vi "SetUpExperiment.vi"(8 "ErrorIn(No Error)":errorcluster caption="entrée d'erreur (pas d'erreur)", 10 "ScanTreeIn":refnum<vi>, 11 "Exper.lvclass":refnum<class "Experiment.lvclass">) -> (0 "sortie d'erreur":errorcluster, 3 "Exper.lvclass Out":refnum<class "Experiment.lvclass">)   [LabVIEW 2019, in "Experiment.lvclass"]
uses:
  Experiment.lvclass
  SetUpExperStates.ctl
  Experiment.lvclass/Experiment.ctl
  DevicesClass/BaseDevice/BaseDevice.lvclass
panel:
  out "MvDir(Up:T)":bool
  out "ScanTag":string
  out "CellPart":T1(ring)
  out "DblClickLine":i32
  in  "ActMeas":bool[](array[boolean])
  in  "ShowParamSuff":bool caption="Show Param. Suffix"
  in  "Param. Suffix":string
  in  "Show2ndScnParNm":bool caption="Show 2nd Scan Param. Name"
  in  "Scan Suffix":string
  in  "ShowScnSuff":bool caption="Show Scan Suffix"
  in  "Display Name":string
  in  "ShowInstrNm":bool caption="Show Instrument Name"
  in  "Before Wait(ms)":u32
  in  "ApplyWait":bool
  in  "Synch":bool
  in  "After Wait(ms)":u32
  in  "TimeMultiple(ms)":u32
  in  "RemFunc":bool
  in  "MoveFuncDown":bool
  in  "AddFunc":bool
  in  "MoveFuncUp":bool
  in  "stop":bool
  in  "FuncPannel":T2(tab)
  in  "ScanFunc":string(tree) caption="Scan Functions"
  in  "MeasFunc":i32(listbox) caption="Measurements Instruments"
  in  "HeaderFunc":i32(listbox) caption="Header Functions"
  in  "PanFunc":i32(listbox) caption="Functions Panels"
  in  "MenuPanels":i32(listbox)
  in  "LoadedDev":string(tree) caption="Loaded Instruments"
  # "Device Parameters"
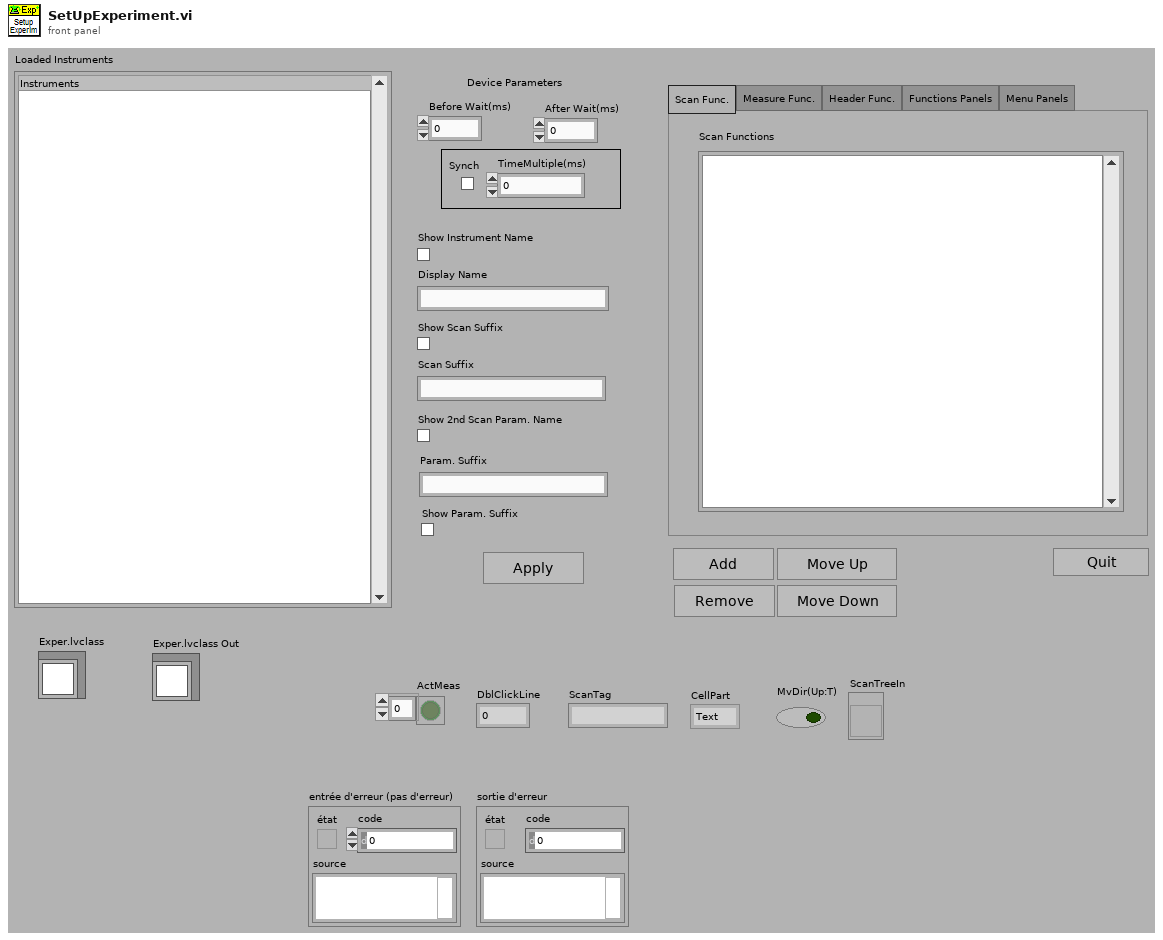
[diagram p1: front panel]
types:
  T1 = enum16{"Text", "Background", "Item Symbol", "Open/Close Symbol", "Hierarchy Lines", "Right Border", "Bottom Border", "Bottom Right Corner", "Unknown Part"}
  T2 = enum32{"Scan Func.", "Measure Func.", "Header Func.", "Functions Panels", "Menu Panels"}
  T3 = typedef "SetUpExperStates.ctl" = enum16{"InitProg", "AddScanFunc", "RmveScanFunc", "PlaceScanFunc", "NewScanTask", "MvScanFunc", "AddMeasFunc", "RmveMeasFunc", "MvMeasFuncUp", "MvMeasFuncDn", "AddHeaderFunc", "RmveHeadFunc", "MvHeadFuncUp", "MvHeadFuncDn", "AddFuncPan", "RemFuncPan", "MvFuncPanUp", "MvFuncPanDn", "AddMenuPan", "RemMenuPan", "Wait", "Stop", "DblClickMeasPan", "DblClickScanPan"}
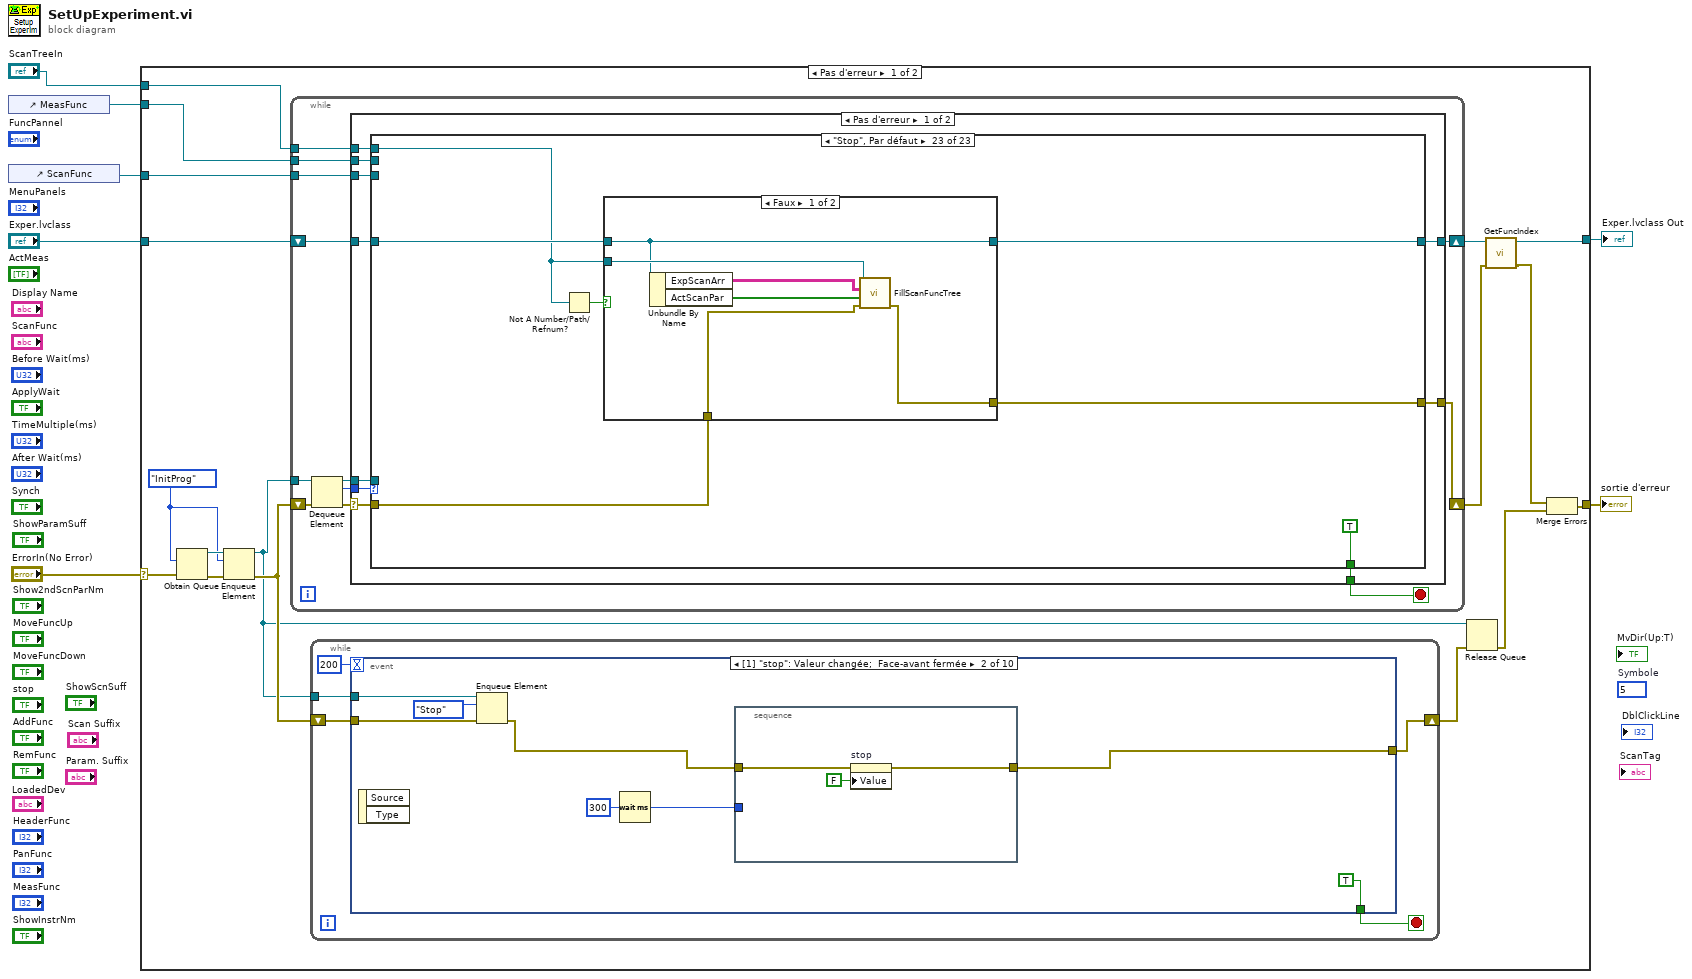
[diagram p0: block diagram]
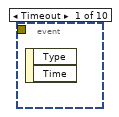
[diagram p2: hidden frame]
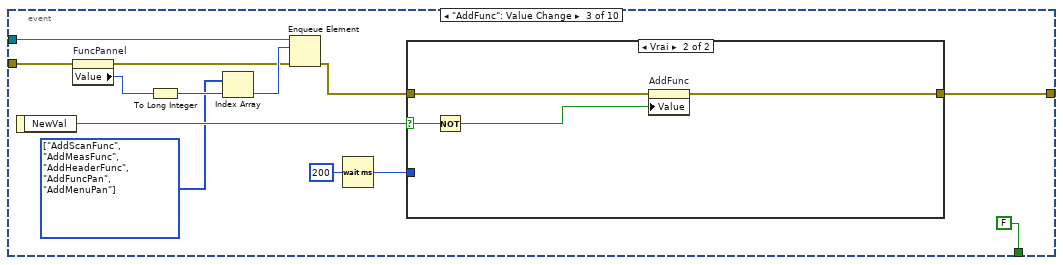
[diagram p3: hidden frame]
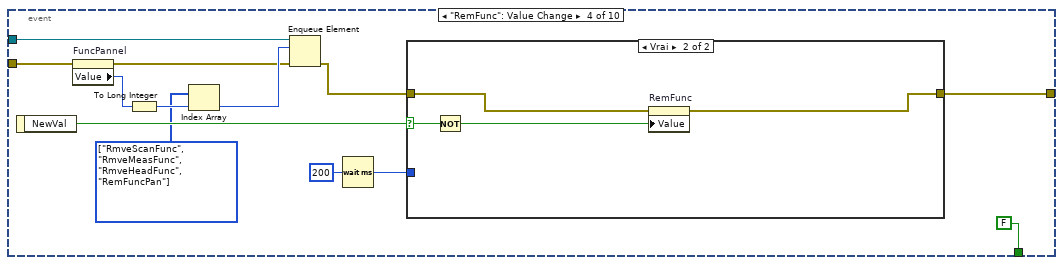
[diagram p5: hidden frame]
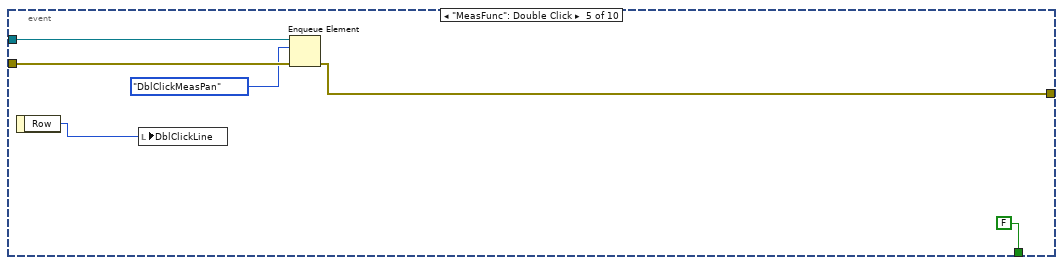
[diagram p7: hidden frame]
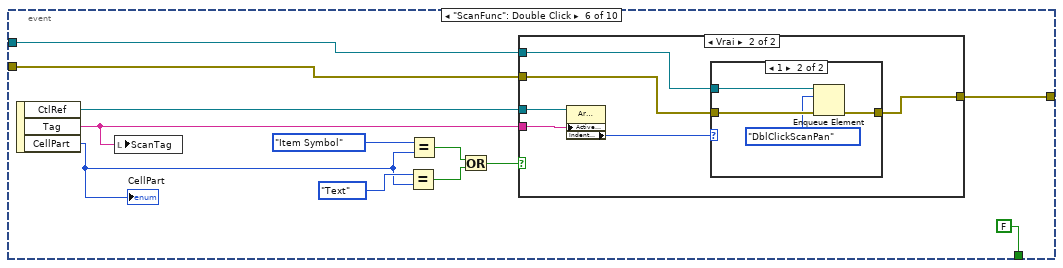
[diagram p8: hidden frame]
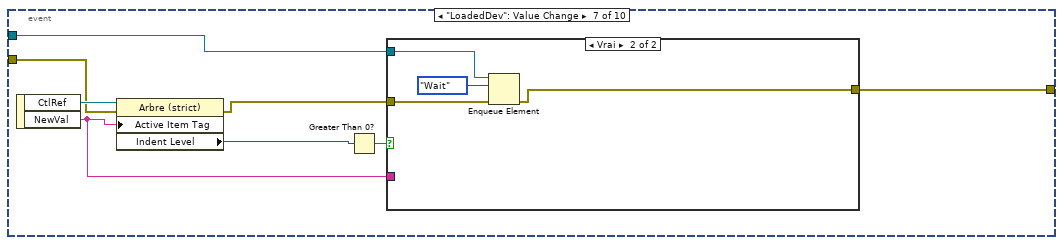
[diagram p11: hidden frame]
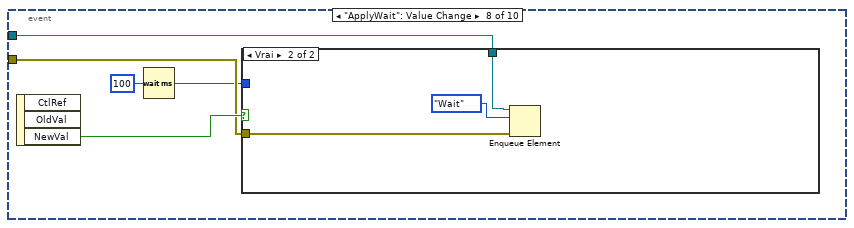
[diagram p13: hidden frame]
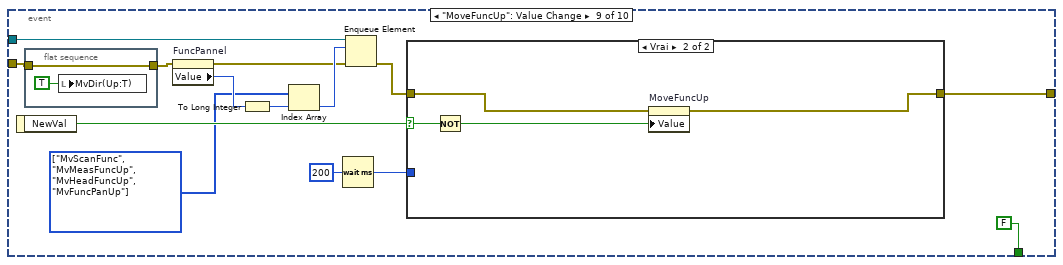
[diagram p15: hidden frame]
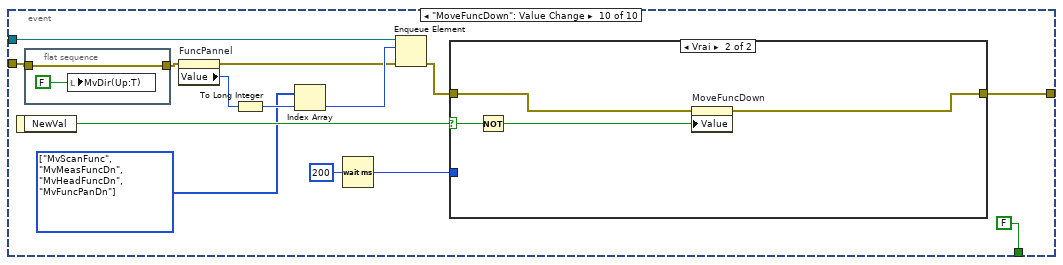
[diagram p17: hidden frame]
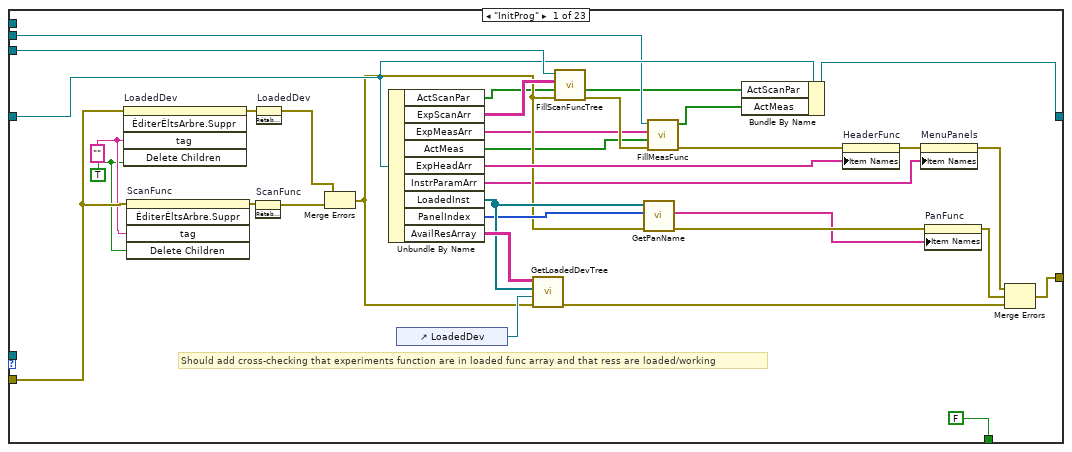
[diagram p19: hidden frame]
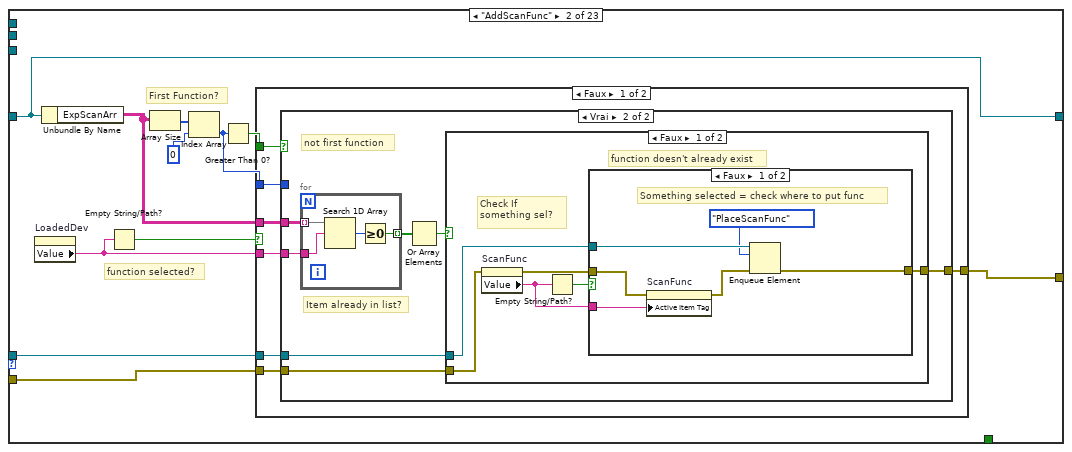
[diagram p20: hidden frame]
diagram:
  (unwired) 5  # Symbole
  n1 = control-ref of="MeasFunc"() -> (w2:refnum<vi>)
  n2 = control-ref of="ScanFunc"() -> (w5:refnum<vi>)
  n3 = case shown="Pas d'erreur" "ErrorIn(No Error)" {
    selector: "ErrorIn(No Error)" -> [w22 w1018]
    tunnel: [w12 w1018] -> w6
    tunnel: w5 -> [w18 _]
    tunnel: "Exper.lvclass" -> [w16 w1017]
    tunnel: [w10 w1017] -> w3
    tunnel: w2 -> [w9 _]
    tunnel: "ScanTreeIn" -> [w8 _]
    frame No Error {
      w21 = SetUpExperStates."InitProg" ("Énum")
      n4 = Obtain Queue(element data type=w21, error in (no error)=w22) -> (queue out=w23:refnum<queue>, error out=w24:errorcluster)  [unwired: 3 in, 1 out]
      n5 = Enqueue Element(queue=w23, element=w21, error in (no error)=w24) -> (queue out=w17:refnum<queue>, error out=w19:errorcluster)  [unwired: 1 in, 1 out]
      n6 = while {
        tunnel: w17 -> [w179]
        shift-right: [w172] -> w14
        shift-left: w19 -> [w177]
        tunnel: w18 -> [w175]
        shift-right: [w173] -> w15
        shift-left: w16 -> [w174]
        tunnel: w9 -> [w171]
        tunnel: w8 -> [w170]
        stop <- w176 stop-if-true
        n7 = Dequeue Element(queue=w179, error in (no error)=w177) -> (queue out=w178:refnum<queue>, element=w180:T3, error out=w181:errorcluster)  [unwired: 1 in, 1 out]
        n8 = case shown="Pas d'erreur" w181 {
          selector: w181 -> [w189 w1015]
          tunnel: w180 -> [w191 _]
          tunnel: w178 -> [w190 _]
          tunnel: [w188 TRUE] -> w176
          tunnel: [w187 w1015] -> w172
          tunnel: w175 -> [w186 _]
          tunnel: w174 -> [w185 w1014]
          tunnel: [w184 w1014] -> w173
          tunnel: w171 -> [w183 _]
          tunnel: w170 -> [w182 _]
          frame No Error {
            n9 = case shown="\"Stop\", Par défaut" w191 {
              tunnel: w190 -> [_ w231 _ _ _ _ _ _ _ _ _ _ _ _ _ _ _ _ _ _ _ _ _]
              tunnel: w189 -> [w206 w230 w290 w308 w390 w421 w471 w513 w536 w552 w582 w611 w646 w683 w709 w730 w763 w822 w880 w906 w936 w965 w1003]
              tunnel: [FALSE _ _ _ _ _ _ _ _ _ _ _ _ _ _ _ _ _ _ _ _ _ TRUE] -> w188
              tunnel: [w222 w234 w284 w301 w384 w418 w469 w512 w535 w546 w577 w609 w644 w682 w704 w738 w761 w820 w879 w901 w935 w961 w1001] -> w187
              tunnel: w186 -> [w218 _ w285 w299 w388 w419 _ _ _ w555 _ _ _ _ _ _ _ _ _ _ _ _ _]
              tunnel: w185 -> [w213 w226 w283 w298 w386 w417 w464 w507 w544 w557 w576 w603 w639 w677 w703 w733 w760 w819 w874 w900 w928 w957 w1004]
              tunnel: [w195 w226 w282 w297 w385 w416 w463 w506 w543 w556 w575 w602 w638 w676 w702 w732 w759 w818 w873 w899 w927 w956 w1000] -> w184
              tunnel: w183 -> [w196 _ _ _ _ _ _ w505 w539 _ w573 w599 _ _ _ _ _ _ _ _ _ _ _]
              tunnel: w182 -> [_ _ _ _ _ _ _ _ _ _ _ _ _ _ _ _ _ _ _ _ _ _ w999]
              frame "InitProg" {
                w205 = "" ("Tag")
                w204 = TRUE ("Supprimer les enfants ?")
                # "Should add cross-checking that experiments function are in loaded func array and that ress are loaded/working"
                n10 = invoke on="LoadedDev" class="Arbre (strict)" method="ÉditerÉltsArbre.Suppr"(error in=w206, "tag"=w205, "Delete Children"=w204) -> (error out=w225:errorcluster)  [unwired: 2 in, 4 out]
                n11 = invoke on="ScanFunc" class="Arbre (strict)" method="ÉditerÉltsArbre.Suppr"(error in=w206, "tag"=w205, "Delete Children"=w204) -> (error out=w221:errorcluster)  [unwired: 2 in, 4 out]
                n12 = invoke on="ScanFunc" class="Arbre (strict)" method="RétablirValParDéfaut"(error in=w221) -> (error out=w219:errorcluster)  [unwired: 2 in, 2 out]
                n13 = invoke on="LoadedDev" class="Arbre (strict)" method="RétablirValParDéfaut"(error in=w225) -> (error out=w220:errorcluster)  [unwired: 2 in, 2 out]
                n14 = Merge Errors(w220, w219) -> (w209:errorcluster)
                n15 = Unbundle By Name(w213) -> ("ActScanPar"=w193:bool[], "ExpScanArr"=w216:string[][], "ExpMeasArr"=w198:string[], "ActMeas"=w197:bool[], "ExpHeadArr"=w217:string[], "InstrParamArr"=w202:string[], "LoadedInst"=w211:refnum<class "BaseDevice.lvclass">[], "PanelIndex"=w210:i32[], "AvailResArray"=w212:string[][])
                n16 = control-ref of="LoadedDev"() -> (w215:refnum<vi>)
                n17 = call "GetLoadedDevTree.vi"("ErrorIn"=w209, "TreeRefIn"=w215, "LoadedInst"=w211, "AvailRessArray"=w212) -> ("ErrorOut"=w223:errorcluster)  [unwired: 7 in]
                n18 = call "FillScanFuncTree.vi"("ErrorIn(No Error)"=w209, "Active ScanPar"=w193, "ScanFunc"=w216, "ScanTreeRef"=w218) -> ("sortie d'erreur"=w200:errorcluster, "Active ScanParOut"=w192:bool[])  [unwired: 6 in]
                n19 = call "GetPanName.vi"("error in (no error)"=w209, "PanelIndex"=w210, "LoadedDev In"=w211) -> ("error out"=w208:errorcluster, "PanelNames"=w207:string[])  [unwired: 6 in, 1 out]
                n20 = call "FillMeasFunc.vi"("ErrorIn(No Error)"=w200, "ActMeas"=w197, "MeasFunc"=w198, "ListRef"=w196) -> ("sortie d'erreur"=w199:errorcluster, "ActMeasOut"=w194:bool[])  [unwired: 6 in]
                n21 = Bundle By Name(cluster=w213, "ActScanPar"=w192, "ActMeas"=w194) -> (w195:refnum<class "Experiment.lvclass">)
                n22 = property on="HeaderFunc" class="LstDér (strict)"(error in=w199, "Item Names"=w217) -> (error out=w203:errorcluster)  [unwired: 1 in, 1 out]
                n23 = property on="MenuPanels" class="LstDér (strict)"(error in=w203, "Item Names"=w202) -> (error out=w201:errorcluster)  [unwired: 1 in, 1 out]
                n24 = property on="PanFunc" class="LstDér (strict)"(error in=w208, "Item Names"=w207) -> (error out=w214:errorcluster)  [unwired: 1 in, 1 out]
                n25 = Merge Errors(w201, w214, w223) -> (w222:errorcluster)
              }
              frame "AddScanFunc" {
                # "function selected?"
                # "First Function?"
                n26 = property on="LoadedDev" class="Arbre (strict)"() -> ("Value"=w229:string)  [unwired: 2 in, 2 out]
                n27 = Unbundle By Name(w226) -> ("ExpScanArr"=w227:string[][])
                n28 = Empty String/Path?(string/path=w229) -> (empty?=w228:bool)
                n29 = Array Size(array=w227) -> (size(s)=w236:i32[])
                n30 = Index Array(array=w236, index=0 ("indice")) -> (element=w232:i32)
                n31 = Greater Than 0?(x=w232) -> (x > 0?=w233:bool)
                n32 = case shown="Faux" w228 {
                  tunnel: [w243 _] -> w234
                  tunnel: w233 -> [w242 _]
                  tunnel: w232 -> [w241 _]
                  tunnel: w231 -> [w240 _]
                  tunnel: w230 -> [w239 _]
                  tunnel: w227 -> [w238 _]
                  tunnel: w229 -> [w237 _]
                  frame False {
                    n33 = case shown="Vrai" w242 {
                      tunnel: [w244 w250] -> w243
                      tunnel: w241 -> [_ _]
                      tunnel: w238 -> [_ w254]
                      tunnel: w237 -> [_ w253]
                      tunnel: w240 -> [w246 w251]
                      tunnel: w239 -> [w245 w248]
                      frame False {
                        # "first function"
                        n34 = Enqueue Element(queue=w246, element=SetUpExperStates."NewScanTask" ("Énum"), error in (no error)=w245) -> (error out=w244:errorcluster)  [unwired: 1 in, 2 out]
                      }
                      frame True {
                        # "not first function"
                        # "Item already in list?"
                        n35 = for {
                          tunnel: [w275] -> w252 mode=indexing
                          tunnel: w253 -> [w274]
                          tunnel: w254 -> [w273] mode=indexing
                          n36 = Search 1D Array(1D array=w273, element=w274) -> (index of element=w276:i32)  [unwired: 1 in]
                          n37 = Greater Or Equal To 0?(x=w276) -> (x >= 0?=w275:bool)
                        }
                        n38 = Or Array Elements(Boolean array=w252) -> (logical OR=w249:bool)
                        n39 = case shown="Faux" w249 {
                          tunnel: w251 -> [w260 _]
                          tunnel: [w259 w271] -> w250
                          tunnel: w248 -> [w256 w271]
                          frame False {
                            # "function doesn't already exist"
                            # "Check If something sel?"
                            n40 = property on="ScanFunc" class="Arbre (strict)"(error in=w256) -> (error out=w255:errorcluster, "Value"=w257:string)  [unwired: 1 in, 1 out]
                            n41 = Empty String/Path?(string/path=w257) -> (empty?=w258:bool)
                            n42 = case shown="Faux" w258 {
                              tunnel: w260 -> [w266 w269]
                              tunnel: [w265 w268] -> w259
                              tunnel: w257 -> [w264 _]
                              tunnel: w255 -> [w262 w267]
                              frame False {
                                # "Something selected = check where to put func"
                                n43 = property on="ScanFunc" class="Arbre (strict)"(error in=w262, "Active Item Tag"=w264) -> (error out=w261:errorcluster)  [unwired: 1 in, 1 out]
                                n44 = Enqueue Element(queue=w266, element=SetUpExperStates."PlaceScanFunc" ("Énum"), error in (no error)=w261) -> (error out=w265:errorcluster)  [unwired: 1 in, 2 out]
                              }
                              frame True {
                                # "Nothing sel = add new Group"
                                n45 = Enqueue Element(queue=w269, element=SetUpExperStates."NewScanTask" ("Énum"), error in (no error)=w267) -> (error out=w268:errorcluster)  [unwired: 1 in, 2 out]
                              }
                            }
                          }
                          frame True {
                            # "function already exist"
                            n46 = One Button Dialog(message="Cette fonction est déjà dans la liste") -> ()  [unwired: 1 in, 1 out]
                          }
                        }
                      }
                    }
                  }
                  frame True {
                    # "No function selected"
                    n47 = One Button Dialog(message="Vous devez sélectionner une fonction à ajouter") -> ()  [unwired: 1 in, 1 out]
                  }
                }
              }
              frame "NewScanTask" {
                n48 = property on="LoadedDev" class="Arbre (strict)"(error in=w290) -> (error out=w286:errorcluster, "Value"=w288:string)  [unwired: 1 in, 1 out]
                n49 = Unbundle By Name(w283) -> ("ExpScanArr"=w289:string[][], "ActScanPar"=w280:bool[])
                n50 = Build Array(w288) -> (w287:string[])
                n51 = Insert Into Array(array=w280, new element=TRUE ("nouvel élément/sous-tableau")) -> (w278:bool[])  [unwired: 1 in]
                n52 = Insert Into Array(array=w289, new element=w287) -> (w281:string[][])  [unwired: 2 in]
                n53 = call "FillScanFuncTree.vi"("ErrorIn(No Error)"=w286, "Active ScanPar"=w278, "ScanFunc"=w281, "ScanTreeRef"=w285) -> ("sortie d'erreur"=w284:errorcluster)  [unwired: 6 in, 1 out]
                n54 = Bundle By Name(cluster=w283, "ExpScanArr"=w281, "ActScanPar"=w278) -> (w282:refnum<class "Experiment.lvclass">)
              }
              frame "PlaceScanFunc" {
                n55 = property on="ScanFunc" class="Arbre (strict)"(error in=w308) -> (error out=w293:errorcluster, "Indent Level"=w306:i32, "Active Item Row Number"=w305:i32, "Active Item Tag"=w304:string)  [unwired: 1 in, 1 out]
                n56 = Unbundle By Name(w298) -> ("ActScanPar"=w296:bool[], "ExpScanArr"=w303:string[][])
                n57 = call <userlib>:"ArrayTo1DString.vi"("ErrorIn(No Error)"=w293, "DelArrEnd(F)"=TRUE ("DelArrEnd"), "tableau"=w303) -> ("sortie d'erreur"=w292:errorcluster, "Array Out"=w294:string[])  [unwired: 6 in, 1 out]
                n58 = Greater Than 0?(x=w306) -> (x > 0?=w307:bool)
                n59 = case shown="Faux" w307 {
                  tunnel: w292 -> [w320 w346]
                  tunnel: [w314 w349] -> w302
                  tunnel: w305 -> [_ w352]
                  tunnel: w304 -> [w321 w351]
                  tunnel: w299 -> [_ w359]
                  tunnel: w303 -> [w315 w347]
                  tunnel: [w313 w350] -> w300
                  tunnel: w296 -> [w311 w345]
                  tunnel: [w310 w344] -> w295
                  tunnel: w294 -> [w309 w343]
                  frame False {
                    # "add function at end of task"
                    # "a parent was selected"
                    n60 = Scan From String(format string="Scan Task_%d" ("chaîne de format"), input string=w321, error in=w320, default 1=0) -> (error out=w319:errorcluster, output 1=w312:i32)  [unwired: 1 in, 2 out]
                    n61 = property on="LoadedDev" class="Arbre (strict)"(error in=w319) -> (error out=w314:errorcluster, "Value"=w316:string)  [unwired: 1 in, 1 out]
                    n62 = for {
                      tunnel: w315 -> [w327] mode=indexing
                      tunnel: w312 -> [w328]
                      tunnel: [w326] -> w313 mode=indexing
                      tunnel: w316 -> [w325]
                      shift-right: [w323] -> w310
                      shift-left: w311 -> [w324]
                      tunnel: w309 -> [w322]
                      i -> [w330]
                      n63 = Equal?(x=w328, y=w330) -> (x = y?=w329:bool)
                      n64 = case shown="Vrai" w329 {
                        tunnel: w327 -> [w332 w337]
                        tunnel: [w332 w341] -> w326
                        tunnel: w325 -> [_ w342]
                        tunnel: w324 -> [w331 w334]
                        tunnel: [w331 w333] -> w323
                        tunnel: w322 -> [_ w335]
                        frame False {
                        }
                        frame True {
                          n65 = Delete From Array(array=w337) -> (deleted portion=w336:string)  [unwired: 2 in, 1 out]
                          n66 = Insert Into Array(array=w337, new element=w342) -> (w341:string[])  [unwired: 1 in]
                          n67 = Search 1D Array(1D array=w335, element=w336) -> (index of element=w339:i32)  [unwired: 1 in]
                          n68 = Increment(x=w339) -> (x+1=w340:i32)
                          n69 = Insert Into Array(array=w334, index=w340, new element=TRUE ("nouvel élément/sous-tableau")) -> (w333:bool[])
                        }
                      }
                    }
                  }
                  frame True {
                    # "add function after task position"
                    # "a child was selected"
                    n70 = call <userlib>:"GetParentTag.vi"("ErrorIn(No Error)"=w346, "LineNum"=w352, "Tag"=w351, "TreeRef"=w359) -> ("sortie d'erreur"=w356:errorcluster, "Parent"=w348:string)  [unwired: 4 in, 2 out]
                    n71 = Scan From String(format string="Scan Task_%d" ("chaîne de format"), input string=w348, error in=w356, default 1=0) -> (error out=w354:errorcluster, output 1=w355:i32)  [unwired: 1 in, 2 out]
                    n72 = property on="LoadedDev" class="Arbre (strict)"(error in=w354) -> (error out=w349:errorcluster, "Value"=w353:string)  [unwired: 1 in, 1 out]
                    n73 = for {
                      tunnel: w347 -> [w366] mode=indexing
                      tunnel: w355 -> [w367]
                      tunnel: [w365] -> w350 mode=indexing
                      tunnel: w353 -> [w364]
                      tunnel: w351 -> [w363]
                      shift-right: [w361] -> w344
                      shift-left: w345 -> [w362]
                      tunnel: w343 -> [w360]
                      i -> [w369]
                      n74 = Equal?(x=w367, y=w369) -> (x = y?=w368:bool)
                      n75 = case shown="Vrai" w368 {
                        tunnel: w366 -> [w371 w379]
                        tunnel: [w371 w381] -> w365
                        tunnel: w364 -> [_ w383]
                        tunnel: w363 -> [_ w377]
                        tunnel: w360 -> [_ w378]
                        tunnel: w362 -> [w370 w376]
                        tunnel: [w370 w375] -> w361
                        frame False {
                        }
                        frame True {
                          n76 = Search 1D Array(1D array=w379, element=w377) -> (index of element=w382:i32)  [unwired: 1 in]
                          n77 = Search 1D Array(1D array=w378, element=w377) -> (index of element=w374:i32)  [unwired: 1 in]
                          n78 = Increment(x=w382) -> (x+1=w380:i32)
                          n79 = Insert Into Array(array=w379, index=w380, new element=w383) -> (w381:string[])
                          n80 = Increment(x=w374) -> (x+1=w373:i32)
                          n81 = Insert Into Array(array=w376, index=w373, new element=TRUE ("nouvel élément/sous-tableau")) -> (w375:bool[])
                        }
                      }
                    }
                  }
                }
                n82 = Bundle By Name(cluster=w298, "ActScanPar"=w295, "ExpScanArr"=w300) -> (w297:refnum<class "Experiment.lvclass">)
                n83 = call "FillScanFuncTree.vi"("ErrorIn(No Error)"=w302, "ScanFunc"=w300, "ScanTreeRef"=w299) -> ("sortie d'erreur"=w301:errorcluster)  [unwired: 7 in, 1 out]
              }
              frame "RmveScanFunc" {
                n84 = property on="ScanFunc" class="Arbre (strict)"(error in=w390) -> (error out=w389:errorcluster, "Value"=w387:string)  [unwired: 1 in, 1 out]
                n85 = Empty String/Path?(string/path=w387) -> (empty?=w391:bool)
                n86 = case shown="Faux" w391 {
                  tunnel: w387 -> [w404 _]
                  tunnel: w389 -> [w397 w414]
                  tunnel: w388 -> [w411 _]
                  tunnel: w386 -> [w407 w413]
                  tunnel: [w412 w413] -> w385
                  tunnel: [w406 w414] -> w384
                  frame False {
                    # "Task Selected?"
                    n87 = Unbundle By Name(w407) -> ("LoadedFuncArr"=w405:string[], "LoadedInst"=w395:refnum<class "BaseDevice.lvclass">[], "ScanSubPan"=w396:refnum<vi>, "ExpScanArr"=w401:string[][], "ActScanPar"=w393:bool[])
                    n88 = Scan From String(format string="Scan Task_%d" ("chaîne de format"), input string=w404, error in=w397) -> (error out=w398:errorcluster, output 1=w403:i32)  [unwired: 2 in, 2 out]
                    n89 = Unbundle By Name(w398) -> ("status"=w402:bool)
                    n90 = call "RemoveScanFunc.vi"("LoadedInstIn"=w395, "LoadedFuncArr"=w405, "ScanFunc"=w404, "ScanSubPan"=w396, "WholeTask(No:T)"=w402, "ScanFuncArrIn"=w401, "ErrorIn(No Error)"=w397, "ActScanPar"=w393, "TaskIdx"=w403) -> ("LoadedInst"=w394:refnum<class "BaseDevice.lvclass">[], "ScanFuncArrOut"=w400:string[][], "ActScanParOut"=w392:bool[], "sortie d'erreur"=w399:errorcluster)  [unwired: 3 in]
                    n91 = Bundle By Name(cluster=w407, "LoadedInst"=w394, "ExpScanArr"=w400, "ActScanPar"=w392) -> (w412:refnum<class "Experiment.lvclass">)
                    n92 = call "FillScanFuncTree.vi"("ErrorIn(No Error)"=w399, "Active ScanPar"=w392, "ScanFunc"=w400, "ScanTreeRef"=w411) -> ("sortie d'erreur"=w409:errorcluster)  [unwired: 6 in, 1 out]
                    n93 = property on="ScanFunc" class="Arbre (strict)"(error in=w409, "Value"="") -> (error out=w406:errorcluster)  [unwired: 1 in, 1 out]
                  }
                  frame True {
                    # "Nothing selected"
                    n94 = One Button Dialog(message="Veuillez sélectionner une fonction à effacer!") -> ()  [unwired: 1 in, 1 out]
                  }
                }
              }
              frame "MvScanFunc" {
                n95 = property on="ScanFunc" class="Arbre (strict)"(error in=w421) -> (error out=w420:errorcluster, "Value"=w423:string)  [unwired: 1 in, 1 out]
                n96 = Empty String/Path?(string/path=w423) -> (empty?=w422:bool)
                n97 = case shown="Faux" w422 {
                  tunnel: w423 -> [w432 _]
                  tunnel: [w434 w459] -> w418
                  tunnel: w420 -> [w436 w459]
                  tunnel: w419 -> [w433 _]
                  tunnel: w417 -> [w428 w458]
                  tunnel: [w427 w458] -> w416
                  frame False {
                    # "Task Selected?"
                    n98 = local read "MvDir(Up:T)"() -> (w424:bool)
                    n99 = Unbundle By Name(w428) -> ("ExpScanArr"=w438:string[][], "ActScanPar"=w426:bool[])
                    n100 = Scan From String(format string="Scan Task_%d" ("chaîne de format"), input string=w432, error in=w436) -> (error out=w435:errorcluster, output 1=w429:i32)  [unwired: 2 in, 2 out]
                    n101 = case shown="Pas d'erreur" w435 {
                      selector: w435 -> [w442 w456]
                      tunnel: w438 -> [w441 w457]
                      tunnel: w432 -> [_ w454]
                      tunnel: [w448 w453] -> w431
                      tunnel: [w444 w452] -> w430
                      tunnel: w429 -> [w440 _]
                      tunnel: w426 -> [w447 w451]
                      tunnel: [w446 w450] -> w425
                      tunnel: w424 -> [w439 w449]
                      frame No Error {
                        # "Move whole task"
                        n102 = call "MoveScanTask.vi"("ActScanPar"=w447, "ErrorIn(No Error)"=w442, "ScanFuncArrIn"=w441, "Dir(Up:T)"=w439, "TaskIdx"=w440) -> ("sortie d'erreur"=w443:errorcluster, "ScanFuncArrOut"=w444:string[][], "ScanFuncOut"=w445:string, "ActScanParOut"=w446:bool[])  [unwired: 3 in]
                        n103 = property on="ScanFunc" class="Arbre (strict)"(error in=w443, "Value"=w445) -> (error out=w448:errorcluster)  [unwired: 1 in, 1 out]
                      }
                      frame Error {
                        n104 = call <vilib>:"Clear Errors.vi"("error in (no error)"=w456) -> ("error out"=w455:errorcluster)  [unwired: 5 in, 1 out]
                        n105 = call "MoveScanFunc.vi"("ActScanPar"=w451, "ErrorIn(No Error)"=w455, "ScanFuncIn"=w457, "Dir(Up:T)"=w449, "Value"=w454) -> ("sortie d'erreur"=w453:errorcluster, "ScanFuncOut"=w452:string[][], "ActScanParOut"=w450:bool[])  [unwired: 4 in]
                      }
                    }
                    n106 = Bundle By Name(cluster=w428, "ExpScanArr"=w430, "ActScanPar"=w425) -> (w427:refnum<class "Experiment.lvclass">)
                    n107 = call "FillScanFuncTree.vi"("ErrorIn(No Error)"=w431, "Active ScanPar"=w425, "ScanFunc"=w430, "ScanTreeRef"=w433) -> ("sortie d'erreur"=w434:errorcluster)  [unwired: 6 in, 1 out]
                  }
                  frame True {
                    # "Nothing selected"
                    n108 = One Button Dialog(message="Veuillez sélectionner une fonction à déplacer!") -> ()  [unwired: 1 in, 1 out]
                  }
                }
              }
              frame "AddMeasFunc" {
                n109 = property on="LoadedDev" class="Arbre (strict)"(error in=w471) -> (error out=w465:errorcluster, "Value"=w462:string)  [unwired: 1 in, 1 out]
                n110 = Unbundle By Name(w464) -> ("ExpMeasArr"=w468:string[], "ActMeas"=w461:bool[])
                n111 = Search 1D Array(1D array=w468, element=w462) -> (index of element=w467:i32)  [unwired: 1 in]
                n112 = Empty String/Path?(string/path=w462) -> (empty?=w470:bool)
                n113 = Greater Or Equal To 0?(x=w467) -> (x >= 0?=w466:bool)
                n114 = case shown="Faux" w470 {
                  tunnel: w465 -> [w478 w503]
                  tunnel: [w479 w502] -> w469
                  tunnel: w462 -> [w476 _]
                  tunnel: w464 -> [w475 w501]
                  tunnel: w468 -> [w477 _]
                  tunnel: w466 -> [w481 _]
                  tunnel: [w474 w501] -> w463
                  tunnel: w462 -> [w473 _]
                  tunnel: w461 -> [w472 _]
                  frame False {
                    n115 = case shown="Vrai" w481 {
                      tunnel: [TRUE ("T button?") w499] -> w480
                      frame False {
                        # "not found"
                      }
                      frame True {
                        n116 = Two Button Dialog(message="Cette fonction existe déjà dans la liste! L'ajouter quand même?") -> (T button?=w499:bool)  [unwired: 2 in]
                      }
                    }
                    n117 = case shown="Vrai" w480 {
                      tunnel: [w483 w497] -> w479
                      tunnel: w478 -> [w483 w492]
                      tunnel: w477 -> [_ w496]
                      tunnel: w476 -> [_ w488]
                      tunnel: w475 -> [w482 w495]
                      tunnel: [w482 w494] -> w474
                      tunnel: w473 -> [_ w489]
                      tunnel: w472 -> [_ w487]
                      frame False {
                      }
                      frame True {
                        n118 = property on="MeasFunc" class="LstDér (strict)"(error in=w492) -> (error out=w484:errorcluster, "Item Names"=w490:string[])  [unwired: 1 in, 1 out]
                        n119 = Insert Into Array(array=w496, new element=w488) -> (w493:string[])  [unwired: 1 in]
                        n120 = Insert Into Array(array=w490, new element=w489) -> (w491:string[])  [unwired: 1 in]
                        n121 = Insert Into Array(array=w487, new element=TRUE ("nouvel élément/sous-tableau")) -> (w485:bool[])  [unwired: 1 in]
                        n122 = property on="MeasFunc" class="LstDér (strict)"(error in=w484, "Item Names"=w491) -> (error out=w497:errorcluster)  [unwired: 1 in, 1 out]
                        n123 = Bundle By Name(cluster=w495, "ExpMeasArr"=w493, "ActMeas"=w485) -> (w494:refnum<class "Experiment.lvclass">)
                      }
                    }
                  }
                  frame True {
                    n124 = call <vilib>:"Clear Errors.vi"("error in (no error)"=w503) -> ("error out"=w502:errorcluster)  [unwired: 5 in, 1 out]
                    n125 = One Button Dialog(message="Vous devez sélectionner une fonction") -> ()  [unwired: 1 in, 1 out]
                  }
                }
              }
              frame "RmveMeasFunc" {
                n126 = property on="MeasFunc" class="LstDér (strict)"(error in=w513) -> (error out=w511:errorcluster, "Item Names"=w510:string[], "Value"=w509:i32)  [unwired: 1 in, 1 out]
                n127 = Greater Or Equal To 0?(x=w509) -> (x >= 0?=w508:bool)
                n128 = case shown="Vrai" w508 {
                  tunnel: [FALSE ("T button?") w532] -> w514
                  frame False {
                    n129 = One Button Dialog(message="Vous devez sélectionner une fonction!") -> ()  [unwired: 1 in, 1 out]
                  }
                  frame True {
                    n130 = Two Button Dialog(message="Retirer cette fonction de la liste de mesures?") -> (T button?=w532:bool)  [unwired: 2 in]
                  }
                }
                n131 = case shown="Vrai" w514 {
                  tunnel: w507 -> [w516 w529]
                  tunnel: w509 -> [_ w519]
                  tunnel: [w516 w526] -> w506
                  tunnel: [w515 w522] -> w512
                  tunnel: w511 -> [w515 w523]
                  tunnel: w510 -> [_ w525]
                  tunnel: w505 -> [_ w517]
                  frame False {
                  }
                  frame True {
                    w521 = 1 ("longueur")
                    n132 = Unbundle By Name(w529) -> ("ExpMeasArr"=w528:string[], "ActMeas"=w520:bool[])
                    n133 = Delete From Array(array=w528, length=w521, index=w519) -> (array with subset deleted=w527:string[])  [unwired: 1 out]
                    n134 = Delete From Array(array=w520, length=w521, index=w519) -> (array with subset deleted=w518:bool[])  [unwired: 1 out]
                    n135 = Delete From Array(array=w525, length=w521, index=w519) -> (array with subset deleted=w524:string[])  [unwired: 1 out]
                    n136 = Bundle By Name(cluster=w529, "ExpMeasArr"=w527, "ActMeas"=w518) -> (w526:refnum<class "Experiment.lvclass">)
                    n137 = call "FillMeasFunc.vi"("ErrorIn(No Error)"=w523, "ActMeas"=w518, "MeasFunc"=w524, "ListRef"=w517) -> ("sortie d'erreur"=w522:errorcluster)  [unwired: 6 in, 1 out]
                  }
                }
              }
              frame "DblClickMeasPan" {
                n138 = local read "DblClickLine"() -> (w542:i32)
                n139 = Unbundle By Name(w544) -> ("ActMeas"=w537:bool[], "ExpMeasArr"=w538:string[])
                n140 = Index Array(array=w537, index=w542) -> (element=w541:bool)
                n141 = Not(x=w541) -> (.not. x?=w540:bool)
                n142 = Replace Array Subset(array=w537, new element=w540, index=w542) -> (w534:bool[])
                n143 = call "FillMeasFunc.vi"("ErrorIn(No Error)"=w536, "ActMeas"=w534, "MeasFunc"=w538, "ListRef"=w539) -> ("sortie d'erreur"=w535:errorcluster)  [unwired: 6 in, 1 out]
                n144 = Bundle By Name(cluster=w544, "ActMeas"=w534) -> (w543:refnum<class "Experiment.lvclass">)
              }
              frame "DblClickScanPan" {
                n145 = Unbundle By Name(w557) -> ("ActScanPar"=w549:bool[], "ExpScanArr"=w554:string[][])
                n146 = local read "ScanTag"() -> (w550:string)
                n147 = call <userlib>:"ArrayTo1DString.vi"("ErrorIn(No Error)"=w552, "DelArrEnd(F)"=TRUE ("DelArrEnd"), "tableau"=w554) -> ("sortie d'erreur"=w547:errorcluster, "Array Out"=w551:string[])  [unwired: 6 in, 1 out]
                n148 = Search 1D Array(1D array=w551, element=w550) -> (index of element=w548:i32)  [unwired: 1 in]
                n149 = Greater Or Equal To 0?(x=w548) -> (x >= 0?=w545:bool)
                n150 = case shown="Vrai" w545 {
                  tunnel: w557 -> [w559 w572]
                  tunnel: [w559 w571] -> w556
                  tunnel: w555 -> [_ w570]
                  tunnel: w549 -> [_ w566]
                  tunnel: w548 -> [_ w565]
                  tunnel: w547 -> [w558 w562]
                  tunnel: [w558 w560] -> w546
                  frame False {
                  }
                  frame True {
                    n151 = Index Array(array=w566, index=w565) -> (element=w567:bool)
                    n152 = Not(x=w567) -> (.not. x?=w563:bool)
                    n153 = Replace Array Subset(array=w566, new element=w563, index=w565) -> (w564:bool[])
                    n154 = Select(t=38, s=w563, f=37) -> (s? t:f=w561:i32)
                    n155 = Bundle By Name(cluster=w572, "ActScanPar"=w564) -> (w571:refnum<class "Experiment.lvclass">)
                    n156 = property class="Arbre (strict)"(reference=w570, error in=w562, "Glyph"=w561) -> (error out=w560:errorcluster)  [unwired: 1 out]
                  }
                }
              }
              frame "MvMeasFuncUp" {
                n157 = property on="MeasFunc" class="LstDér (strict)"(error in=w582) -> (error out=w580:errorcluster, "Value"=w579:i32)  [unwired: 1 in, 1 out]
                n158 = Unbundle By Name(w576) -> ("ExpMeasArr"=w581:string[], "ActMeas"=w574:bool[])
                n159 = Greater Than 0?(x=w579) -> (x > 0?=w578:bool)
                n160 = case shown="Vrai" w578 {
                  tunnel: w576 -> [w584 w598]
                  tunnel: w581 -> [_ w592]
                  tunnel: w579 -> [_ w588]
                  tunnel: w580 -> [w583 w585]
                  tunnel: [w584 w597] -> w575
                  tunnel: [w583 w596] -> w577
                  tunnel: w574 -> [_ w587]
                  tunnel: w573 -> [_ w594]
                  frame False {
                    # "already at top"
                  }
                  frame True {
                    n161 = call <userlib>:"ShiftArrElStringGen.vi"("ErrorIn(No Error)"=w585, "Index"=w588, "Array In"=w592) -> ("sortie d'erreur"=w589:errorcluster, "NewIndex"=w590:i32, "Array Out"=w591:string[])  [unwired: 6 in]
                    n162 = call <userlib>:"ShiftArrElBoolGen.vi"("ErrorIn(No Error)"=w585, "Index"=w588, "Array In"=w587) -> ("Array Out"=w586:bool[])  [unwired: 6 in, 2 out]
                    n163 = call "FillMeasFunc.vi"("ErrorIn(No Error)"=w589, "ActMeas"=w586, "MeasFunc"=w591, "ListRef"=w594) -> ("sortie d'erreur"=w595:errorcluster, "ActMeasOut"=w593:bool[])  [unwired: 6 in]
                    n164 = Bundle By Name(cluster=w598, "ExpMeasArr"=w591, "ActMeas"=w593) -> (w597:refnum<class "Experiment.lvclass">)
                    n165 = property on="MeasFunc" class="LstDér (strict)"(error in=w595, "Value"=w590) -> (error out=w596:errorcluster)  [unwired: 1 in, 1 out]
                  }
                }
              }
              frame "MvMeasFuncDn" {
                n166 = Unbundle By Name(w603) -> ("ExpMeasArr"=w608:string[], "ActMeas"=w600:bool[])
                n167 = property on="MeasFunc" class="LstDér (strict)"(error in=w611) -> (error out=w610:errorcluster, "Value"=w606:i32, "Item Names"=w601:string[])  [unwired: 1 in, 1 out]
                n168 = Array Size(array=w608) -> (size(s)=w607:i32)
                n169 = Increment(x=w606) -> (x+1=w605:i32)
                n170 = Equal?(x=w607, y=w605) -> (x = y?=w604:bool)
                n171 = case shown="Faux" w604 {
                  tunnel: w603 -> [w634 w636]
                  tunnel: w608 -> [w632 _]
                  tunnel: w606 -> [w618 _]
                  tunnel: w610 -> [w617 w635]
                  tunnel: [w628 w636] -> w602
                  tunnel: [w627 w635] -> w609
                  tunnel: w601 -> [w624 _]
                  tunnel: w600 -> [w622 _]
                  tunnel: w599 -> [w613 _]
                  frame False {
                    w619 = 1 ("longueur")
                    n172 = Delete From Array(array=w632, length=1 ("longueur"), index=w618) -> (deleted portion=w630:string[], array with subset deleted=w631:string[])
                    n173 = Delete From Array(array=w622, length=w619, index=w618) -> (deleted portion=w623:bool[], array with subset deleted=w621:bool[])
                    n174 = Increment(x=w618) -> (x+1=w620:i32)
                    n175 = Delete From Array(array=w624, length=w619, index=w618) -> (deleted portion=w626:string[], array with subset deleted=w625:string[])
                    n176 = Insert Into Array(array=w631, index=w620, new element=w630) -> (w629:string[])
                    n177 = Insert Into Array(array=w621, index=w620, new element=w623) -> (w614:bool[])
                    n178 = Insert Into Array(array=w625, index=w620, new element=w626) -> (w612:string[])
                    n179 = call "FillMeasFunc.vi"("ErrorIn(No Error)"=w617, "ActMeas"=w614, "MeasFunc"=w612, "ListRef"=w613) -> ("sortie d'erreur"=w616:errorcluster, "ActMeasOut"=w615:bool[])  [unwired: 6 in]
                    n180 = Bundle By Name(cluster=w634, "ExpMeasArr"=w629, "ActMeas"=w615) -> (w628:refnum<class "Experiment.lvclass">)
                    n181 = property on="MeasFunc" class="LstDér (strict)"(error in=w616, "Value"=w620) -> (error out=w627:errorcluster)  [unwired: 1 in, 1 out]
                  }
                  frame True {
                    # "already at bottom"
                  }
                }
              }
              frame "AddHeaderFunc" {
                n182 = property on="LoadedDev" class="Arbre (strict)"(error in=w646) -> (error out=w640:errorcluster, "Value"=w637:string)  [unwired: 1 in, 1 out]
                n183 = Unbundle By Name(w639) -> ("ExpHeadArr"=w643:string[])
                n184 = Empty String/Path?(string/path=w637) -> (empty?=w645:bool)
                n185 = Search 1D Array(1D array=w643, element=w637) -> (index of element=w642:i32)  [unwired: 1 in]
                n186 = Greater Or Equal To 0?(x=w642) -> (x >= 0?=w641:bool)
                n187 = case shown="Faux" w645 {
                  tunnel: w640 -> [w652 w674]
                  tunnel: [w653 w673] -> w644
                  tunnel: w637 -> [w650 _]
                  tunnel: w639 -> [w649 w672]
                  tunnel: w643 -> [w651 _]
                  tunnel: w641 -> [w655 _]
                  tunnel: [w648 w672] -> w638
                  tunnel: w637 -> [w647 _]
                  frame False {
                    n188 = case shown="Vrai" w655 {
                      tunnel: [TRUE ("T button?") FALSE] -> w654
                      frame False {
                      }
                      frame True {
                        n189 = One Button Dialog(message="Cette fonction existe déjà dans la liste! Inutile de duppliquer!") -> ()  [unwired: 1 in, 1 out]
                      }
                    }
                    n190 = case shown="Vrai" w654 {
                      tunnel: [w657 w668] -> w653
                      tunnel: w652 -> [w657 w662]
                      tunnel: w651 -> [_ w667]
                      tunnel: w650 -> [_ w666]
                      tunnel: w649 -> [w656 w665]
                      tunnel: [w656 w664] -> w648
                      tunnel: w647 -> [_ w659]
                      frame False {
                      }
                      frame True {
                        n191 = property on="HeaderFunc" class="LstDér (strict)"(error in=w662) -> (error out=w658:errorcluster, "Item Names"=w660:string[])  [unwired: 1 in, 1 out]
                        n192 = Insert Into Array(array=w667, new element=w666) -> (w663:string[])  [unwired: 1 in]
                        n193 = Insert Into Array(array=w660, new element=w659) -> (w661:string[])  [unwired: 1 in]
                        n194 = Bundle By Name(cluster=w665, "ExpHeadArr"=w663) -> (w664:refnum<class "Experiment.lvclass">)
                        n195 = property on="HeaderFunc" class="LstDér (strict)"(error in=w658, "Item Names"=w661) -> (error out=w668:errorcluster)  [unwired: 1 in, 1 out]
                      }
                    }
                  }
                  frame True {
                    n196 = call <vilib>:"Clear Errors.vi"("error in (no error)"=w674) -> ("error out"=w673:errorcluster)  [unwired: 5 in, 1 out]
                    n197 = One Button Dialog(message="Vous devez sélectionner une fonction") -> ()  [unwired: 1 in, 1 out]
                  }
                }
              }
              frame "RmveHeadFunc" {
                n198 = property on="HeaderFunc" class="LstDér (strict)"(error in=w683) -> (error out=w681:errorcluster, "Item Names"=w680:string[], "Value"=w679:i32)  [unwired: 1 in, 1 out]
                n199 = Greater Or Equal To 0?(x=w679) -> (x >= 0?=w678:bool)
                n200 = case shown="Vrai" w678 {
                  tunnel: [FALSE ("T button?") w699] -> w684
                  frame False {
                    n201 = One Button Dialog(message="Vous devez sélectionner une fonction!") -> ()  [unwired: 1 in, 1 out]
                  }
                  frame True {
                    n202 = Two Button Dialog(message="Retirer cette fonction de la liste?") -> (T button?=w699:bool)  [unwired: 2 in]
                  }
                }
                n203 = case shown="Vrai" w684 {
                  tunnel: w677 -> [w686 w696]
                  tunnel: w679 -> [_ w692]
                  tunnel: [w686 w693] -> w676
                  tunnel: [w685 w687] -> w682
                  tunnel: w681 -> [w685 w688]
                  tunnel: w680 -> [_ w689]
                  frame False {
                  }
                  frame True {
                    w691 = 1 ("longueur")
                    n204 = Unbundle By Name(w696) -> ("ExpHeadArr"=w695:string[])
                    n205 = Delete From Array(array=w695, length=w691, index=w692) -> (array with subset deleted=w694:string[])  [unwired: 1 out]
                    n206 = Delete From Array(array=w689, length=w691, index=w692) -> (array with subset deleted=w690:string[])  [unwired: 1 out]
                    n207 = property on="HeaderFunc" class="LstDér (strict)"(error in=w688, "Item Names"=w690) -> (error out=w687:errorcluster)  [unwired: 1 in, 1 out]
                    n208 = Bundle By Name(cluster=w696, "ExpHeadArr"=w694) -> (w693:refnum<class "Experiment.lvclass">)
                  }
                }
              }
              frame "MvHeadFuncUp" {
                n209 = property on="HeaderFunc" class="LstDér (strict)"(error in=w709) -> (error out=w707:errorcluster, "Value"=w706:i32, "Item Names"=w701:string[])  [unwired: 1 in, 1 out]
                n210 = Unbundle By Name(w703) -> ("ExpHeadArr"=w708:string[])
                n211 = Greater Than 0?(x=w706) -> (x > 0?=w705:bool)
                n212 = case shown="Vrai" w705 {
                  tunnel: w703 -> [w711 w727]
                  tunnel: w708 -> [_ w725]
                  tunnel: w706 -> [_ w714]
                  tunnel: w707 -> [w710 w722]
                  tunnel: [w711 w720] -> w702
                  tunnel: [w710 w719] -> w704
                  tunnel: w701 -> [_ w715]
                  frame False {
                    # "already at top"
                  }
                  frame True {
                    n213 = Delete From Array(array=w725, length=1 ("longueur"), index=w714) -> (deleted portion=w723:string[], array with subset deleted=w724:string[])
                    n214 = Delete From Array(array=w715, length=1 ("longueur"), index=w714) -> (deleted portion=w718:string[], array with subset deleted=w717:string[])
                    n215 = Decrement(x=w714) -> (x-1=w713:i32)
                    n216 = Insert Into Array(array=w724, index=w713, new element=w723) -> (w721:string[])
                    n217 = Insert Into Array(array=w717, index=w713, new element=w718) -> (w712:string[])
                    n218 = Bundle By Name(cluster=w727, "ExpHeadArr"=w721) -> (w720:refnum<class "Experiment.lvclass">)
                    n219 = property on="HeaderFunc" class="LstDér (strict)"(error in=w722, "Item Names"=w712, "Value"=w713) -> (error out=w719:errorcluster)  [unwired: 1 in, 1 out]
                  }
                }
              }
              frame "MvHeadFuncDn" {
                n220 = Unbundle By Name(w733) -> ("ExpHeadArr"=w737:string[])
                n221 = property on="HeaderFunc" class="LstDér (strict)"(error in=w730) -> (error out=w731:errorcluster, "Value"=w729:i32, "Item Names"=w728:string[])  [unwired: 1 in, 1 out]
                n222 = Array Size(array=w737) -> (size(s)=w736:i32)
                n223 = Increment(x=w729) -> (x+1=w735:i32)
                n224 = Equal?(x=w736, y=w735) -> (x = y?=w734:bool)
                n225 = case shown="Faux" w734 {
                  tunnel: w733 -> [w754 w756]
                  tunnel: w737 -> [w752 _]
                  tunnel: w729 -> [w741 _]
                  tunnel: [w748 w756] -> w732
                  tunnel: [w747 w755] -> w738
                  tunnel: w731 -> [w746 w755]
                  tunnel: w728 -> [w742 _]
                  frame False {
                    n226 = Delete From Array(array=w752, length=1 ("longueur"), index=w741) -> (deleted portion=w750:string[], array with subset deleted=w751:string[])
                    n227 = Increment(x=w741) -> (x+1=w739:i32)
                    n228 = Delete From Array(array=w742, length=1 ("longueur"), index=w741) -> (deleted portion=w745:string[], array with subset deleted=w744:string[])
                    n229 = Insert Into Array(array=w751, index=w739, new element=w750) -> (w749:string[])
                    n230 = Insert Into Array(array=w744, index=w739, new element=w745) -> (w740:string[])
                    n231 = Bundle By Name(cluster=w754, "ExpHeadArr"=w749) -> (w748:refnum<class "Experiment.lvclass">)
                    n232 = property on="HeaderFunc" class="LstDér (strict)"(error in=w746, "Item Names"=w740, "Value"=w739) -> (error out=w747:errorcluster)  [unwired: 1 in, 1 out]
                  }
                  frame True {
                    # "already at bottom"
                  }
                }
              }
              frame "AddFuncPan" {
                n233 = property on="LoadedDev" class="Arbre (strict)"(error in=w763) -> (error out=w757:errorcluster, "Value"=w758:string)  [unwired: 1 in, 1 out]
                n234 = Empty String/Path?(string/path=w758) -> (empty?=w762:bool)
                n235 = case shown="Faux" w762 {
                  tunnel: w757 -> [w770 w814]
                  tunnel: [w775 w813] -> w761
                  tunnel: w758 -> [w767 _]
                  tunnel: w760 -> [w773 w812]
                  tunnel: [w774 w812] -> w759
                  frame False {
                    n236 = Unbundle By Name(w773) -> ("ExpPanArr"=w766:string[], "LoadedInst"=w772:refnum<class "BaseDevice.lvclass">[], "LoadedFuncArr"=w771:string[])
                    n237 = call "CheckFuncPan.vi"("error in (no error)"=w770, "Function"=w767, "LoadedFuncArr"=w771, "LoadedInst"=w772) -> ("error out"=w769:errorcluster, "PanelName"=w765:string, "OperCanceled"=w768:bool, "LoadedInst Out"=w764:refnum<class "BaseDevice.lvclass">[])  [unwired: 4 in]
                    n238 = case shown="Faux" w768 {
                      tunnel: [w789 w810] -> w775
                      tunnel: [w788 w811] -> w774
                      tunnel: w773 -> [w786 w811]
                      tunnel: w766 -> [w780 _]
                      tunnel: w769 -> [w779 w810]
                      tunnel: w765 -> [w784 _]
                      tunnel: w767 -> [w781 _]
                      tunnel: w764 -> [w776 _]
                      frame False {
                        n239 = property on="PanFunc" class="LstDér (strict)"(error in=w779) -> (error out=w777:errorcluster, "Item Names"=w778:string[])  [unwired: 1 in, 1 out]
                        n240 = Search 1D Array(1D array=w778, element=w784) -> (index of element=w782:i32)  [unwired: 1 in]
                        n241 = Greater Or Equal To 0?(x=w782) -> (x >= 0?=w783:bool)
                        n242 = case shown="Faux" w783 {
                          tunnel: [TRUE ("T button?") FALSE] -> w790
                          tunnel: w784 -> [w791 _]
                          tunnel: [w792 _] -> w787
                          tunnel: [w791 _] -> w785
                          tunnel: w781 -> [w792 _]
                          frame False {
                          }
                          frame True {
                            n243 = One Button Dialog(message="Cette fonction existe déjà dans la liste! Inutile de duppliquer!") -> ()  [unwired: 1 in, 1 out]
                          }
                        }
                        n244 = case shown="Vrai" w790 {
                          tunnel: [w797 w809] -> w789
                          tunnel: w777 -> [w797 w804]
                          tunnel: w780 -> [_ w808]
                          tunnel: w786 -> [w796 w807]
                          tunnel: [w796 w806] -> w788
                          tunnel: w785 -> [_ w801]
                          tunnel: w787 -> [_ w800]
                          tunnel: w776 -> [_ w798]
                          frame False {
                          }
                          frame True {
                            n245 = property on="PanFunc" class="LstDér (strict)"(error in=w804) -> (error out=w799:errorcluster, "Item Names"=w802:string[])  [unwired: 1 in, 1 out]
                            n246 = Insert Into Array(array=w808, new element=w800) -> (w805:string[])  [unwired: 1 in]
                            n247 = Insert Into Array(array=w802, new element=w801) -> (w803:string[])  [unwired: 1 in]
                            n248 = Bundle By Name(cluster=w807, "LoadedInst"=w798, "ExpPanArr"=w805) -> (w806:refnum<class "Experiment.lvclass">)
                            n249 = property on="PanFunc" class="LstDér (strict)"(error in=w799, "Item Names"=w803) -> (error out=w809:errorcluster)  [unwired: 1 in, 1 out]
                          }
                        }
                      }
                      frame True {
                        # "operation canceled"
                      }
                    }
                  }
                  frame True {
                    n250 = call <vilib>:"Clear Errors.vi"("error in (no error)"=w814) -> ("error out"=w813:errorcluster)  [unwired: 5 in, 1 out]
                    n251 = One Button Dialog(message="Vous devez sélectionner une fonction") -> ()  [unwired: 1 in, 1 out]
                  }
                }
              }
              frame "AddMenuPan" {
                n252 = property on="LoadedDev" class="Arbre (strict)"(error in=w822) -> (error out=w816:errorcluster, "Value"=w817:string)  [unwired: 1 in, 1 out]
                n253 = Empty String/Path?(string/path=w817) -> (empty?=w821:bool)
                n254 = case shown="Faux" w821 {
                  tunnel: w816 -> [w832 w871]
                  tunnel: [w836 w870] -> w820
                  tunnel: w817 -> [w830 _]
                  tunnel: w819 -> [w834 w869]
                  tunnel: [w835 w869] -> w818
                  frame False {
                    n255 = Unbundle By Name(w834) -> ("InstrParamArr"=w829:string[], "LoadedInst"=w833:refnum<class "BaseDevice.lvclass">[], "LoadedFuncArr"=w823:string[], "ParamIndex 2"=w824:i32[])
                    n256 = call "CheckMenuPan.vi"("error in (no error)"=w832, "Function"=w830, "LoadedFuncArr"=w823, "LoadedInst"=w833) -> ("error out"=w831:errorcluster, "PanelName"=w828:string, "MenuPanInstrInd"=w825:i32, "LoadedInst Out"=w827:refnum<class "BaseDevice.lvclass">[], "OperCanceled"=w826:bool)  [unwired: 3 in]
                    n257 = case shown="Faux" w826 {
                      tunnel: [w849 w867] -> w836
                      tunnel: [w848 w868] -> w835
                      tunnel: w834 -> [w847 w868]
                      tunnel: w829 -> [w845 _]
                      tunnel: w831 -> [w844 w867]
                      tunnel: w828 -> [w838 _]
                      tunnel: w827 -> [w841 _]
                      tunnel: w825 -> [w840 _]
                      tunnel: w824 -> [w837 _]
                      frame False {
                        n258 = property on="MenuPanels" class="LstDér (strict)"(error in=w844) -> (error out=w842:errorcluster, "Item Names"=w843:string[])  [unwired: 1 in, 1 out]
                        n259 = Search 1D Array(1D array=w843, element=w838) -> (index of element=w846:i32)  [unwired: 1 in]
                        n260 = Greater Or Equal To 0?(x=w846) -> (x >= 0?=w839:bool)
                        n261 = case shown="Faux" w839 {
                          tunnel: [w863 w866] -> w849
                          tunnel: w842 -> [w858 w866]
                          tunnel: w845 -> [w862 _]
                          tunnel: w847 -> [w861 w865]
                          tunnel: [w860 w865] -> w848
                          tunnel: w838 -> [w851 _]
                          tunnel: w841 -> [w854 _]
                          tunnel: w840 -> [w853 _]
                          tunnel: w837 -> [w850 _]
                          frame False {
                            n262 = Insert Into Array(array=w850, new element=w853) -> (w852:i32[])  [unwired: 1 in]
                            n263 = property on="MenuPanels" class="LstDér (strict)"(error in=w858) -> (error out=w855:errorcluster, "Item Names"=w856:string[])  [unwired: 1 in, 1 out]
                            n264 = Insert Into Array(array=w862, new element=w851) -> (w859:string[])  [unwired: 1 in]
                            n265 = Insert Into Array(array=w856, new element=w851) -> (w857:string[])  [unwired: 1 in]
                            n266 = Bundle By Name(cluster=w861, "LoadedInst"=w854, "ParamIndex 2"=w852, "InstrParamArr"=w859) -> (w860:refnum<class "Experiment.lvclass">)
                            n267 = property on="MenuPanels" class="LstDér (strict)"(error in=w855, "Item Names"=w857) -> (error out=w863:errorcluster)  [unwired: 1 in, 1 out]
                          }
                          frame True {
                            n268 = One Button Dialog(message="Cette fonction existe déjà dans la liste! Inutile de duppliquer!") -> ()  [unwired: 1 in, 1 out]
                          }
                        }
                      }
                      frame True {
                        # "operation canceled"
                      }
                    }
                  }
                  frame True {
                    n269 = call <vilib>:"Clear Errors.vi"("error in (no error)"=w871) -> ("error out"=w870:errorcluster)  [unwired: 5 in, 1 out]
                    n270 = One Button Dialog(message="Vous devez sélectionner une fonction") -> ()  [unwired: 1 in, 1 out]
                  }
                }
              }
              frame "RemFuncPan" {
                n271 = property on="PanFunc" class="LstDér (strict)"(error in=w880) -> (error out=w878:errorcluster, "Item Names"=w877:string[], "Value"=w876:i32)  [unwired: 1 in, 1 out]
                n272 = Greater Or Equal To 0?(x=w876) -> (x >= 0?=w875:bool)
                n273 = case shown="Vrai" w875 {
                  tunnel: [FALSE ("T button?") w896] -> w881
                  frame False {
                    n274 = One Button Dialog(message="Vous devez sélectionner une fonction!") -> ()  [unwired: 1 in, 1 out]
                  }
                  frame True {
                    n275 = Two Button Dialog(message="Retirer cette fonction de la liste?") -> (T button?=w896:bool)  [unwired: 2 in]
                  }
                }
                n276 = case shown="Vrai" w881 {
                  tunnel: w874 -> [w883 w893]
                  tunnel: w876 -> [_ w889]
                  tunnel: [w883 w890] -> w873
                  tunnel: [w882 w884] -> w879
                  tunnel: w878 -> [w882 w885]
                  tunnel: w877 -> [_ w886]
                  frame False {
                  }
                  frame True {
                    w888 = 1 ("longueur")
                    n277 = Unbundle By Name(w893) -> ("ExpPanArr"=w892:string[])
                    n278 = Delete From Array(array=w892, length=w888, index=w889) -> (array with subset deleted=w891:string[])  [unwired: 1 out]
                    n279 = Delete From Array(array=w886, length=w888, index=w889) -> (array with subset deleted=w887:string[])  [unwired: 1 out]
                    n280 = property on="PanFunc" class="LstDér (strict)"(error in=w885, "Item Names"=w887) -> (error out=w884:errorcluster)  [unwired: 1 in, 1 out]
                    n281 = Bundle By Name(cluster=w893, "ExpPanArr"=w891) -> (w890:refnum<class "Experiment.lvclass">)
                  }
                }
              }
              frame "MvFuncPanUp" {
                n282 = property on="PanFunc" class="LstDér (strict)"(error in=w906) -> (error out=w904:errorcluster, "Value"=w903:i32, "Item Names"=w898:string[])  [unwired: 1 in, 1 out]
                n283 = Unbundle By Name(w900) -> ("ExpPanArr"=w905:string[])
                n284 = Greater Than 0?(x=w903) -> (x > 0?=w902:bool)
                n285 = case shown="Vrai" w902 {
                  tunnel: w900 -> [w908 w925]
                  tunnel: w905 -> [_ w923]
                  tunnel: w903 -> [_ w910]
                  tunnel: w904 -> [w907 w920]
                  tunnel: [w908 w917] -> w899
                  tunnel: [w907 w916] -> w901
                  tunnel: w898 -> [_ w911]
                  frame False {
                    # "already at top"
                  }
                  frame True {
                    n286 = Delete From Array(array=w911, length=1 ("longueur"), index=w910) -> (deleted portion=w914:string[], array with subset deleted=w913:string[])
                    n287 = Delete From Array(array=w923, length=1 ("longueur"), index=w910) -> (deleted portion=w921:string[], array with subset deleted=w922:string[])
                    n288 = Decrement(x=w910) -> (x-1=w915:i32)
                    n289 = Decrement(x=w910) -> (x-1=w919:i32)
                    n290 = Insert Into Array(array=w913, index=w915, new element=w914) -> (w909:string[])
                    n291 = Insert Into Array(array=w922, index=w919, new element=w921) -> (w918:string[])
                    n292 = Bundle By Name(cluster=w925, "ExpPanArr"=w918) -> (w917:refnum<class "Experiment.lvclass">)
                    n293 = property on="PanFunc" class="LstDér (strict)"(error in=w920, "Item Names"=w909, "Value"=w919) -> (error out=w916:errorcluster)  [unwired: 1 in, 1 out]
                  }
                }
              }
              frame "MvFuncPanDn" {
                n294 = Unbundle By Name(w928) -> ("ExpPanArr"=w934:string[])
                n295 = property on="PanFunc" class="LstDér (strict)"(error in=w936) -> (error out=w929:errorcluster, "Value"=w932:i32, "Item Names"=w926:string[])  [unwired: 1 in, 1 out]
                n296 = Array Size(array=w934) -> (size(s)=w933:i32)
                n297 = Increment(x=w932) -> (x+1=w931:i32)
                n298 = Equal?(x=w933, y=w931) -> (x = y?=w930:bool)
                n299 = case shown="Faux" w930 {
                  tunnel: w928 -> [w953 w955]
                  tunnel: w934 -> [w951 _]
                  tunnel: w932 -> [w938 _]
                  tunnel: [w946 w955] -> w927
                  tunnel: [w945 w954] -> w935
                  tunnel: w929 -> [w944 w954]
                  tunnel: w926 -> [w939 _]
                  frame False {
                    n300 = Delete From Array(array=w951, length=1 ("longueur"), index=w938) -> (deleted portion=w949:string[], array with subset deleted=w950:string[])
                    n301 = Delete From Array(array=w939, length=1 ("longueur"), index=w938) -> (deleted portion=w942:string[], array with subset deleted=w941:string[])
                    n302 = Increment(x=w938) -> (x+1=w948:i32)
                    n303 = Increment(x=w938) -> (x+1=w943:i32)
                    n304 = Insert Into Array(array=w950, index=w948, new element=w949) -> (w947:string[])
                    n305 = Insert Into Array(array=w941, index=w943, new element=w942) -> (w937:string[])
                    n306 = Bundle By Name(cluster=w953, "ExpPanArr"=w947) -> (w946:refnum<class "Experiment.lvclass">)
                    n307 = property on="PanFunc" class="LstDér (strict)"(error in=w944, "Item Names"=w937, "Value"=w948) -> (error out=w945:errorcluster)  [unwired: 1 in, 1 out]
                  }
                  frame True {
                    # "already at bottom"
                  }
                }
              }
              frame "Wait" {
                n308 = Unbundle By Name(w957) -> ("LoadedInst"=w959:refnum<class "BaseDevice.lvclass">[], "LoadedFuncArr"=w964:string[])
                n309 = property on="LoadedDev" class="Arbre (strict)"(error in=w965) -> (error out=w962:errorcluster, "Value"=w963:string)  [unwired: 1 in, 1 out]
                n310 = Search 1D Array(1D array=w964, element=w963) -> (index of element=w958:i32)  [unwired: 1 in]
                n311 = local read "ApplyWait"() -> (w960:bool)
                n312 = case shown="Vrai" w960 {
                  selector: w960 -> [_ w987]
                  tunnel: w959 -> [w978 w985]
                  tunnel: w962 -> [w970 w983]
                  tunnel: [w974 w979] -> w961
                  tunnel: w958 -> [w971 w984]
                  tunnel: w957 -> [w973 w982]
                  tunnel: [w973 w981] -> w956
                  frame False {
                    n313 = Index Array(array=w978, index=w971) -> (element=w972:refnum<class "BaseDevice.lvclass">)
                    n314 = call "GetWaitValues.vi"("error in (no error)"=w970, "BaseDevice en entrée"=w972) -> ("error out"=w974:errorcluster, "Afterwait(ms)"=w975:u32, "Beforewait(ms)"=w966:u32, "SynchToClk(ms)"=w969:i32)  [unwired: 5 in, 1 out]
                    n315 = Greater Or Equal To 0?(x=w969) -> (x >= 0?=w977:bool)
                    n316 = local write "Before Wait(ms)"(w966) -> ()
                    n317 = local write "After Wait(ms)"(w975) -> ()
                    n318 = local write "Synch"(w977) -> ()
                    n319 = Select(t=w969, s=w977, f=0 ("cas faux")) -> (s? t:f=w976:i32)
                    n320 = To Unsigned Long Integer(number=w976) -> (unsigned 32bit integer=w967:u32)
                    n321 = local write "TimeMultiple(ms)"(w967) -> ()
                  }
                  frame True {
                    n322 = in-place {
                      in-place-border: w983 -> [w997]
                      in-place-border: [w995] -> w979
                      n323 = in-place-array #1(w985, w984) -> (w998:refnum<class "BaseDevice.lvclass">)
                      n324 = local read "TimeMultiple(ms)"() -> (w991:u32)
                      n325 = local read "Synch"() -> (w994:bool)
                      n326 = local read "Before Wait(ms)"() -> (w989:u32)
                      n327 = local read "After Wait(ms)"() -> (w988:u32)
                      n328 = To Long Integer(number=w991) -> (32bit integer=w990:i32)
                      n329 = Select(t=w990, s=w994, f=-1 ("cas faux")) -> (s? t:f=w992:i32)
                      n330 = call "SetWaitValues.vi"("SynchToClk(ms)"=w992, "error in (no error)"=w997, "Afterwait(ms)"=w988, "Beforewait(ms)"=w989, "BaseDevice en entrée"=w998) -> ("error out"=w995:errorcluster, "BaseDevice en sortie"=w996:refnum<class "BaseDevice.lvclass">)  [unwired: 5 in]
                      n331 = in-place-array #1(w996) -> (w980:refnum<class "BaseDevice.lvclass">[])  [unwired: 1 out]
                    }
                    n332 = Not(x=w987) -> (.not. x?=w986:bool)
                    n333 = local write "ApplyWait"(w986) -> ()
                    n334 = Bundle By Name(cluster=w982, "LoadedInst"=w980) -> (w981:refnum<class "Experiment.lvclass">)
                  }
                }
              }
              frame "Stop", Default {
                n335 = Not A Number/Path/Refnum?(number/path/refnum=w999) -> (NaN/Path/Refnum?=w1002:bool)
                n336 = case shown="Faux" w1002 {
                  tunnel: w1004 -> [w1006 w1012]
                  tunnel: w1003 -> [w1010 w1013]
                  tunnel: w999 -> [w1008 _]
                  tunnel: [w1007 w1013] -> w1001
                  tunnel: [w1006 w1012] -> w1000
                  frame False {
                    n337 = Unbundle By Name(w1006) -> ("ExpScanArr"=w1009:string[][], "ActScanPar"=w1011:bool[])
                    n338 = call "FillScanFuncTree.vi"("ErrorIn(No Error)"=w1010, "Active ScanPar"=w1011, "ScanFunc"=w1009, "ScanTreeRef"=w1008) -> ("sortie d'erreur"=w1007:errorcluster)  [unwired: 6 in, 1 out]
                  }
                  frame True {
                  }
                }
              }
            }
          }
          frame Error {
          }
        }
      }
      n339 = while {
        shift-right: [w26] -> w20
        shift-left: w19 -> [w27]
        tunnel: w17 -> [w28]
        stop <- w25 stop-if-true
        n340 = event shown="[1] \"stop\": Valeur changée;  Face-avant fermée" {
          selector: _ -> [_ _ _ _ _ _ _ _ _ _]
          dyn-events: _ -> [_ _ _ _ _ _ _ _ _ _]
          timeout: 200 -> [_ _ _ _ _ _ _ _ _ _]
          tunnel: w28 -> [_ w34 w50 w68 w82 w94 w112 w122 w138 w159]
          tunnel: w27 -> [_ w36 w44 w62 w80 w92 w111 w121 w128 w149]
          tunnel: [_ w37 w52 w70 w78 w91 w109 _ w140 w161] -> w26
          tunnel: [_ TRUE FALSE FALSE FALSE FALSE _ _ FALSE FALSE] -> w25
          event Timeout {
            n341 = event-data() -> ()  [unwired: 1 in, 2 out]
          }
          event "stop": Value Change; Panel Close {
            n342 = event-data() -> ()  [unwired: 1 in, 2 out]
            n343 = Enqueue Element(queue=w34, element=SetUpExperStates."Stop" ("Énum"), error in (no error)=w36) -> (error out=w35:errorcluster)  [unwired: 1 in, 2 out]
            n344 = Wait (ms)(milliseconds to wait=u32 300 ("attente (ms)")) -> (millisecond timer value=w31:u32)
            n345 = stacked-sequence {
              tunnel: [w40] -> w37
              tunnel: w35 -> [w39]
              tunnel: w31 -> [_]
              frame #0 {
                n346 = property on="stop" class="Bool (strict)"(error in=w39, "Value"=FALSE ("stop")) -> (error out=w40:errorcluster)  [unwired: 1 in, 1 out]
              }
            }
          }
          event "AddFunc": Value Change {
            w43 = T3[] [enum."AddScanFunc", enum."AddMeasFunc", enum."AddHeaderFunc", enum."AddFuncPan", enum."AddMenuPan"] items=["InitProg", "AddScanFunc", "RmveScanFunc", "PlaceScanFunc", "NewScanTask", "MvScanFunc", "AddMeasFunc", "RmveMeasFunc", "MvMeasFuncUp", "MvMeasFuncDn", "AddHeaderFunc", "RmveHeadFunc", "MvHeadFuncUp", "MvHeadFuncDn", "AddFuncPan", "RemFuncPan", "MvFuncPanUp", "MvFuncPanDn", "AddMenuPan", "RemMenuPan", "Wait", "Stop", "DblClickMeasPan", "DblClickScanPan"]
            n347 = event-data() -> ("NewVal"=w53:bool)  [unwired: 1 in]
            n348 = property on="FuncPannel" class="Onglet (strict)"(error in=w44) -> (error out=w41:errorcluster, "Value"=w46:T2)  [unwired: 1 in, 1 out]
            n349 = To Long Integer(number=w46) -> (32bit integer=w45:i32)
            n350 = Index Array(array=w43, index=w45) -> (element=w42:T3)
            n351 = Enqueue Element(queue=w50, element=w42, error in (no error)=w41) -> (error out=w51:errorcluster)  [unwired: 1 in, 2 out]
            n352 = Wait (ms)(milliseconds to wait=u32 200 ("attente (ms)")) -> (millisecond timer value=w47:u32)
            n353 = case shown="Vrai" w53 {
              selector: w53 -> [_ w58]
              tunnel: w51 -> [w54 w56]
              tunnel: [w54 w55] -> w52
              tunnel: w47 -> [_ _]
              frame False {
              }
              frame True {
                n354 = Not(x=w58) -> (.not. x?=w57:bool)
                n355 = property on="AddFunc" class="Bool (strict)"(error in=w56, "Value"=w57) -> (error out=w55:errorcluster)  [unwired: 1 in, 1 out]
              }
            }
          }
          event "RemFunc": Value Change {
            w61 = T3[] [enum."RmveScanFunc", enum."RmveMeasFunc", enum."RmveHeadFunc", enum."RemFuncPan"] items=["InitProg", "AddScanFunc", "RmveScanFunc", "PlaceScanFunc", "NewScanTask", "MvScanFunc", "AddMeasFunc", "RmveMeasFunc", "MvMeasFuncUp", "MvMeasFuncDn", "AddHeaderFunc", "RmveHeadFunc", "MvHeadFuncUp", "MvHeadFuncDn", "AddFuncPan", "RemFuncPan", "MvFuncPanUp", "MvFuncPanDn", "AddMenuPan", "RemMenuPan", "Wait", "Stop", "DblClickMeasPan", "DblClickScanPan"]
            n356 = event-data() -> ("NewVal"=w71:bool)  [unwired: 1 in]
            n357 = property on="FuncPannel" class="Onglet (strict)"(error in=w62) -> (error out=w59:errorcluster, "Value"=w64:T2)  [unwired: 1 in, 1 out]
            n358 = To Long Integer(number=w64) -> (32bit integer=w63:i32)
            n359 = Index Array(array=w61, index=w63) -> (element=w60:T3)
            n360 = Enqueue Element(queue=w68, element=w60, error in (no error)=w59) -> (error out=w69:errorcluster)  [unwired: 1 in, 2 out]
            n361 = Wait (ms)(milliseconds to wait=u32 200 ("attente (ms)")) -> (millisecond timer value=w65:u32)
            n362 = case shown="Vrai" w71 {
              selector: w71 -> [_ w76]
              tunnel: w69 -> [w72 w74]
              tunnel: [w72 w73] -> w70
              tunnel: w65 -> [_ _]
              frame False {
              }
              frame True {
                n363 = Not(x=w76) -> (.not. x?=w75:bool)
                n364 = property on="RemFunc" class="Bool (strict)"(error in=w74, "Value"=w75) -> (error out=w73:errorcluster)  [unwired: 1 in, 1 out]
              }
            }
          }
          event "MeasFunc": Double Click {
            n365 = event-data() -> ("Row"=w77:i32)  [unwired: 1 in]
            n366 = local write "DblClickLine"(w77) -> ()
            n367 = Enqueue Element(queue=w82, element=SetUpExperStates."DblClickMeasPan", error in (no error)=w80) -> (error out=w78:errorcluster)  [unwired: 1 in, 2 out]
          }
          event "ScanFunc": Double Click {
            n368 = event-data() -> ("CtlRef"=w84:refnum<vi>, "Tag"=w83:string, "CellPart"=w88:T1)  [unwired: 1 in]
            "CellPart" <- w88
            n369 = local write "ScanTag"(w83) -> ()
            n370 = Equal?(x=T1."Text" ("CellPart"), y=w88) -> (x = y?=w87:bool)
            n371 = Equal?(x=T1."Item Symbol" ("CellPart"), y=w88) -> (x = y?=w86:bool)
            n372 = Or(x=w86, y=w87) -> (x .or. y?=w85:bool)
            n373 = case shown="Vrai" w85 {
              tunnel: w94 -> [_ w101]
              tunnel: w92 -> [w95 w100]
              tunnel: [w95 w99] -> w91
              tunnel: w84 -> [_ w98]
              tunnel: w83 -> [_ w97]
              frame False {
              }
              frame True {
                n374 = property class="Arbre (strict)"(reference=w98, "Active Item Tag"=w97) -> ("Indent Level"=w96:i32)  [unwired: 1 in, 2 out]
                n375 = case shown="1" w96 {
                  tunnel: w101 -> [_ w106]
                  tunnel: w100 -> [w102 w105]
                  tunnel: [w102 w103] -> w99
                  frame 0, Default {
                  }
                  frame 1 {
                    n376 = Enqueue Element(queue=w106, element=SetUpExperStates."DblClickScanPan", error in (no error)=w105) -> (error out=w103:errorcluster)  [unwired: 1 in, 2 out]
                  }
                }
              }
            }
          }
          event "LoadedDev": Value Change {
            n377 = event-data() -> ("CtlRef"=w114:refnum<vi>, "NewVal"=w108:string)  [unwired: 1 in]
            n378 = property class="Arbre (strict)"(reference=w114, error in=w111, "Active Item Tag"=w108) -> (error out=w110:errorcluster, "Indent Level"=w107:i32)  [unwired: 1 out]
            n379 = Greater Than 0?(x=w107) -> (x > 0?=w113:bool)
            n380 = case shown="Vrai" w113 {
              tunnel: w112 -> [_ w119]
              tunnel: w110 -> [w115 w118]
              tunnel: [w115 w117] -> w109
              tunnel: w108 -> [_ _]
              frame False {
              }
              frame True {
                n381 = Enqueue Element(queue=w119, element=SetUpExperStates."Wait" ("élément"), error in (no error)=w118) -> (error out=w117:errorcluster)  [unwired: 1 in, 2 out]
              }
            }
          }
          event "ApplyWait": Value Change {
            n382 = event-data() -> ("NewVal"=w124:bool)  [unwired: 1 in, 2 out]
            n383 = Wait (ms)(milliseconds to wait=u32 100 ("attente (ms)")) -> (millisecond timer value=w120:u32)
            n384 = case shown="Vrai" w124 {
              tunnel: w122 -> [_ w127]
              tunnel: w121 -> [_ w126]
              tunnel: w120 -> [_ _]
              frame False {
              }
              frame True {
                n385 = Enqueue Element(queue=w127, element=SetUpExperStates."Wait" ("Énum"), error in (no error)=w126) -> ()  [unwired: 1 in, 3 out]
              }
            }
          }
          event "MoveFuncUp": Value Change {
            w132 = T3[] [enum."MvScanFunc", enum."MvMeasFuncUp", enum."MvHeadFuncUp", enum."MvFuncPanUp"] items=["InitProg", "AddScanFunc", "RmveScanFunc", "PlaceScanFunc", "NewScanTask", "MvScanFunc", "AddMeasFunc", "RmveMeasFunc", "MvMeasFuncUp", "MvMeasFuncDn", "AddHeaderFunc", "RmveHeadFunc", "MvHeadFuncUp", "MvHeadFuncDn", "AddFuncPan", "RemFuncPan", "MvFuncPanUp", "MvFuncPanDn", "AddMenuPan", "RemMenuPan", "Wait", "Stop", "DblClickMeasPan", "DblClickScanPan"]
            n386 = event-data() -> ("NewVal"=w141:bool)  [unwired: 1 in]
            n387 = flat-sequence {
              tunnel: [w142] -> w129
              tunnel: w128 -> [w142]
              frame #0 {
                n388 = local write "MvDir(Up:T)"(TRUE ("MvDir(Down:F)")) -> ()
              }
            }
            n389 = property on="FuncPannel" class="Onglet (strict)"(error in=w129) -> (error out=w130:errorcluster, "Value"=w134:T2)  [unwired: 1 in, 1 out]
            n390 = To Long Integer(number=w134) -> (32bit integer=w133:i32)
            n391 = Index Array(array=w132, index=w133) -> (element=w131:T3)
            n392 = Wait (ms)(milliseconds to wait=u32 200 ("attente (ms)")) -> (millisecond timer value=w135:u32)
            n393 = Enqueue Element(queue=w138, element=w131, error in (no error)=w130) -> (error out=w139:errorcluster)  [unwired: 1 in, 2 out]
            n394 = case shown="Vrai" w141 {
              selector: w141 -> [_ w148]
              tunnel: w139 -> [w144 w146]
              tunnel: [w144 w145] -> w140
              tunnel: w135 -> [_ _]
              frame False {
              }
              frame True {
                n395 = Not(x=w148) -> (.not. x?=w147:bool)
                n396 = property on="MoveFuncUp" class="Bool (strict)"(error in=w146, "Value"=w147) -> (error out=w145:errorcluster)  [unwired: 1 in, 1 out]
              }
            }
          }
          event "MoveFuncDown": Value Change {
            w153 = T3[] [enum."MvScanFunc", enum."MvMeasFuncDn", enum."MvHeadFuncDn", enum."MvFuncPanDn"] items=["InitProg", "AddScanFunc", "RmveScanFunc", "PlaceScanFunc", "NewScanTask", "MvScanFunc", "AddMeasFunc", "RmveMeasFunc", "MvMeasFuncUp", "MvMeasFuncDn", "AddHeaderFunc", "RmveHeadFunc", "MvHeadFuncUp", "MvHeadFuncDn", "AddFuncPan", "RemFuncPan", "MvFuncPanUp", "MvFuncPanDn", "AddMenuPan", "RemMenuPan", "Wait", "Stop", "DblClickMeasPan", "DblClickScanPan"]
            n397 = event-data() -> ("NewVal"=w162:bool)  [unwired: 1 in]
            n398 = flat-sequence {
              tunnel: [w163] -> w150
              tunnel: w149 -> [w163]
              frame #0 {
                n399 = local write "MvDir(Up:T)"(FALSE ("MvDir(Down:F)")) -> ()
              }
            }
            n400 = property on="FuncPannel" class="Onglet (strict)"(error in=w150) -> (error out=w151:errorcluster, "Value"=w155:T2)  [unwired: 1 in, 1 out]
            n401 = To Long Integer(number=w155) -> (32bit integer=w154:i32)
            n402 = Index Array(array=w153, index=w154) -> (element=w152:T3)
            n403 = Wait (ms)(milliseconds to wait=u32 200 ("attente (ms)")) -> (millisecond timer value=w156:u32)
            n404 = Enqueue Element(queue=w159, element=w152, error in (no error)=w151) -> (error out=w160:errorcluster)  [unwired: 1 in, 2 out]
            n405 = case shown="Vrai" w162 {
              selector: w162 -> [_ w169]
              tunnel: w160 -> [w165 w167]
              tunnel: [w165 w166] -> w161
              tunnel: w156 -> [_ _]
              frame False {
              }
              frame True {
                n406 = Not(x=w169) -> (.not. x?=w168:bool)
                n407 = property on="MoveFuncDown" class="Bool (strict)"(error in=w167, "Value"=w168) -> (error out=w166:errorcluster)  [unwired: 1 in, 1 out]
              }
            }
          }
        }
      }
      n408 = Release Queue(queue=w17, error in (no error)=w20) -> (error out=w13:errorcluster)  [unwired: 1 in, 2 out]
      n409 = call "GetFuncIndex.vi"("error in (no error)"=w14, "Experiment en entrée"=w15) -> ("error out"=w11:errorcluster, "Experiment en sortie"=w10:refnum<class "Experiment.lvclass">)  [unwired: 8 in]
      n410 = Merge Errors(w11, w13) -> (w12:errorcluster)
    }
    frame Error {
    }
  }
  "sortie d'erreur" <- w6
  "Exper.lvclass Out" <- w3
